vi "check_SQL_statement_type.vi"(7 "SQL_statement_type":T1, 8 "error_in":errorcluster, 11 "SQL_statement_in":string) -> (0 "error_out":errorcluster, 3 "SQL_statement_out":string)   [LabVIEW 2020]
uses:
  SQL_statement_type.ctl
  AULocalize/SubVIs/Get Localized Phrase Compact Interface 0D.vi
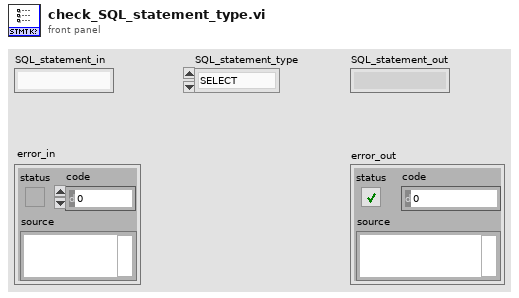
[diagram p1: front panel]
types:
  T1 = typedef "SQL_statement_type.ctl" = enum16{"SELECT", "INSERT", "UPDATE", "DELETE"}
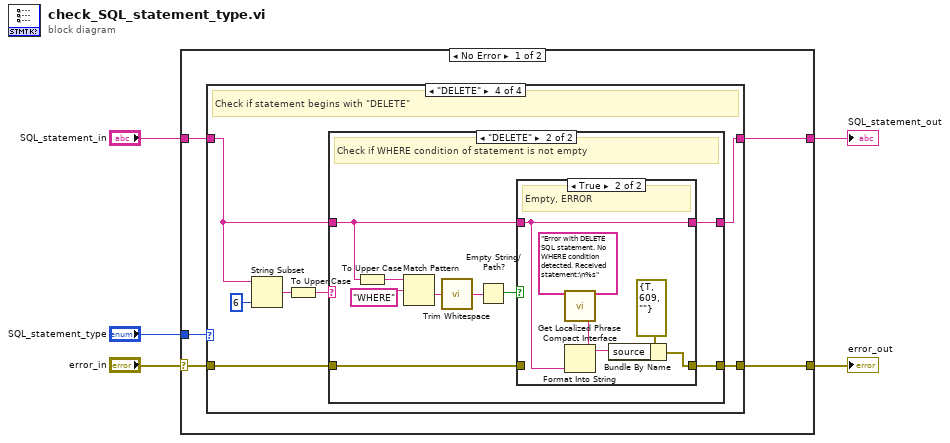
[diagram p0: block diagram]
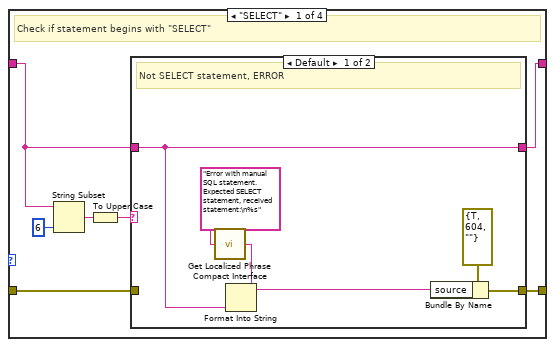
[diagram p2: hidden frame]
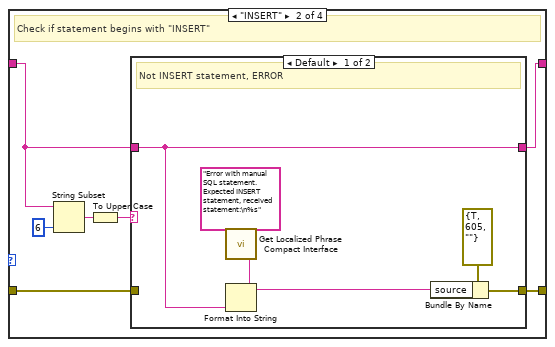
[diagram p4: hidden frame]
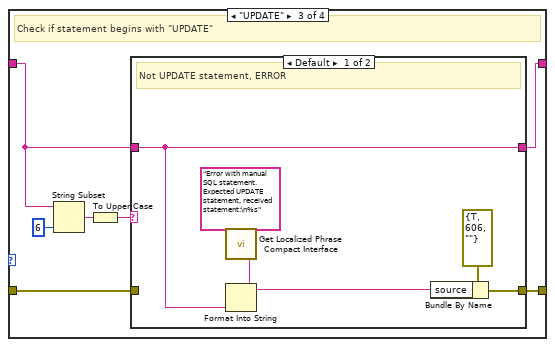
[diagram p6: hidden frame]
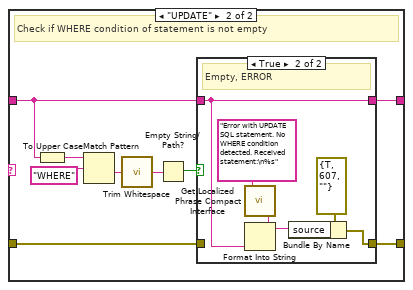
[diagram p7: hidden frame]
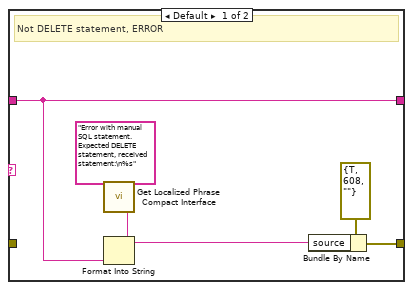
[diagram p9: hidden frame]
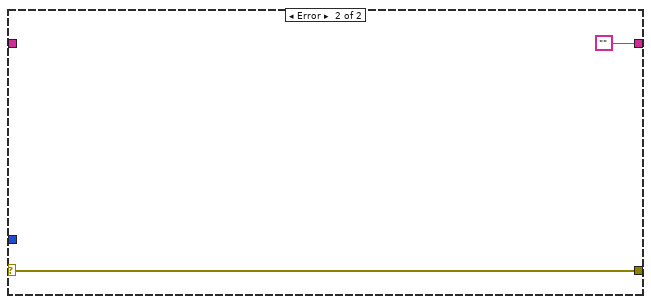
[diagram p11: hidden frame]
diagram:
  n1 = case shown="No Error" "error_in" {
    selector: "error_in" -> [w9 w102]
    tunnel: "SQL_statement_in" -> [w7 _]
    tunnel: [w8 w102] -> w3
    tunnel: "SQL_statement_type" -> [w10 _]
    tunnel: [w6 ""] -> w1
    frame No Error {
      n2 = case shown="\"DELETE\"" w10 {
        tunnel: w7 -> [w14 w29 w44 w74]
        tunnel: w9 -> [w15 w30 w45 w75]
        tunnel: [w16 w31 w46 w76] -> w8
        tunnel: [w11 w26 w41 w71] -> w6
        frame "SELECT" {
          # "Check if statement begins with \"SELECT\""
          n3 = String Subset(string=w14, length (rest)=6 ("length (rest)")) -> (substring=w13:string)  [unwired: 1 in]
          n4 = To Upper Case(1:w13) -> (0:w12:string)
          n5 = case shown="Default" w12 {
            tunnel: [w23 w24] -> w16
            tunnel: w15 -> [_ w24]
            tunnel: w14 -> [w19 w25]
            tunnel: [w19 w25] -> w11
            frame Default {
              # "Not SELECT statement, ERROR"
              n6 = call-poly "Get Localized Phrase Compact Interface.vi"("Key"="Error with manual SQL statement. Expected SELECT statement, received statement:\n%s" ("source")) -> ("Translated Phrase"=w18:string)
              n7 = Format Into String(format string=w18, w19) -> (resulting string=w21:string)  [unwired: 2 in, 1 out]
              n8 = Bundle By Name(cluster=errorcluster {"status"=TRUE, "code"=604, "source"=""} ("error_in"), "source"=w21) -> (w23:errorcluster)
            }
            frame "SELECT" {
              # "SELECT statement, OK"
            }
          }
        }
        frame "INSERT" {
          # "Check if statement begins with \"INSERT\""
          n9 = String Subset(string=w29, length (rest)=6 ("length (rest)")) -> (substring=w28:string)  [unwired: 1 in]
          n10 = To Upper Case(1:w28) -> (0:w27:string)
          n11 = case shown="Default" w27 {
            tunnel: [w38 w39] -> w31
            tunnel: w30 -> [_ w39]
            tunnel: w29 -> [w34 w40]
            tunnel: [w34 w40] -> w26
            frame Default {
              # "Not INSERT statement, ERROR"
              n12 = call-poly "Get Localized Phrase Compact Interface.vi"("Key"="Error with manual SQL statement. Expected INSERT statement, received statement:\n%s" ("source")) -> ("Translated Phrase"=w33:string)
              n13 = Format Into String(format string=w33, w34) -> (resulting string=w36:string)  [unwired: 2 in, 1 out]
              n14 = Bundle By Name(cluster=errorcluster {"status"=TRUE, "code"=605, "source"=""} ("error_in"), "source"=w36) -> (w38:errorcluster)
            }
            frame "INSERT" {
              # "INSERT statement, OK"
            }
          }
        }
        frame "UPDATE" {
          # "Check if statement begins with \"UPDATE\""
          n15 = String Subset(string=w44, length (rest)=6 ("length (rest)")) -> (substring=w43:string)  [unwired: 1 in]
          n16 = To Upper Case(1:w43) -> (0:w42:string)
          n17 = case shown="Default" w42 {
            tunnel: [w53 w56] -> w46
            tunnel: w45 -> [_ w55]
            tunnel: w44 -> [w49 w57]
            tunnel: [w49 w54] -> w41
            frame Default {
              # "Not UPDATE statement, ERROR"
              n18 = call-poly "Get Localized Phrase Compact Interface.vi"("Key"="Error with manual SQL statement. Expected UPDATE statement, received statement:\n%s" ("source")) -> ("Translated Phrase"=w48:string)
              n19 = Format Into String(format string=w48, w49) -> (resulting string=w51:string)  [unwired: 2 in, 1 out]
              n20 = Bundle By Name(cluster=errorcluster {"status"=TRUE, "code"=606, "source"=""} ("error_in"), "source"=w51) -> (w53:errorcluster)
            }
            frame "UPDATE" {
              # "Check if WHERE condition of statement is not empty"
              n21 = To Upper Case(1:w57) -> (0:w60:string)
              n22 = Match Pattern(string=w60, regular expression="WHERE") -> (after substring=w61:string)  [unwired: 1 in, 3 out]
              n23 = call <vilib>:"Trim Whitespace.vi"("string"=w61) -> ("trimmed string"=w59:string)  [unwired: 1 in]
              n24 = Empty String/Path?(string/path=w59) -> (empty?=w58:bool)
              n25 = case shown="True" w58 {
                tunnel: w57 -> [w64 w67]
                tunnel: [w63 w66] -> w56
                tunnel: w55 -> [w63 _]
                tunnel: [w64 w67] -> w54
                frame False {
                  # "Not empty, OK"
                }
                frame True {
                  # "Empty, ERROR"
                  n26 = call-poly "Get Localized Phrase Compact Interface.vi"("Key"="Error with UPDATE SQL statement. No WHERE condition detected. Received statement:\n%s" ("source")) -> ("Translated Phrase"=w65:string)
                  n27 = Format Into String(format string=w65, w67) -> (resulting string=w70:string)  [unwired: 2 in, 1 out]
                  n28 = Bundle By Name(cluster=errorcluster {"status"=TRUE, "code"=607, "source"=""} ("error_in"), "source"=w70) -> (w66:errorcluster)
                }
              }
            }
          }
        }
        frame "DELETE" {
          # "Check if statement begins with \"DELETE\""
          n29 = String Subset(string=w74, length (rest)=6 ("length (rest)")) -> (substring=w73:string)  [unwired: 1 in]
          n30 = To Upper Case(1:w73) -> (0:w72:string)
          n31 = case shown="\"DELETE\"" w72 {
            tunnel: [w83 w86] -> w76
            tunnel: w75 -> [_ w85]
            tunnel: w74 -> [w80 w87]
            tunnel: [w80 w84] -> w71
            frame Default {
              # "Not DELETE statement, ERROR"
              n32 = call-poly "Get Localized Phrase Compact Interface.vi"("Key"="Error with manual SQL statement. Expected DELETE statement, received statement:\n%s" ("source")) -> ("Translated Phrase"=w78:string)
              n33 = Format Into String(format string=w78, w80) -> (resulting string=w81:string)  [unwired: 2 in, 1 out]
              n34 = Bundle By Name(cluster=errorcluster {"status"=TRUE, "code"=608, "source"=""} ("error_in"), "source"=w81) -> (w83:errorcluster)
            }
            frame "DELETE" {
              # "Check if WHERE condition of statement is not empty"
              n35 = To Upper Case(1:w87) -> (0:w90:string)
              n36 = Match Pattern(string=w90, regular expression="WHERE") -> (after substring=w91:string)  [unwired: 1 in, 3 out]
              n37 = call <vilib>:"Trim Whitespace.vi"("string"=w91) -> ("trimmed string"=w89:string)  [unwired: 1 in]
              n38 = Empty String/Path?(string/path=w89) -> (empty?=w88:bool)
              n39 = case shown="True" w88 {
                tunnel: w87 -> [w94 w97]
                tunnel: [w93 w96] -> w86
                tunnel: w85 -> [w93 _]
                tunnel: [w94 w97] -> w84
                frame False {
                  # "Not empty, OK"
                }
                frame True {
                  # "Empty, ERROR"
                  n40 = call-poly "Get Localized Phrase Compact Interface.vi"("Key"="Error with DELETE SQL statement. No WHERE condition detected. Received statement:\n%s" ("source")) -> ("Translated Phrase"=w95:string)
                  n41 = Format Into String(format string=w95, w97) -> (resulting string=w100:string)  [unwired: 2 in, 1 out]
                  n42 = Bundle By Name(cluster=errorcluster {"status"=TRUE, "code"=609, "source"=""} ("error_in"), "source"=w100) -> (w96:errorcluster)
                }
              }
            }
          }
        }
      }
    }
    frame Error {
    }
  }
  "error_out" <- w3
  "SQL_statement_out" <- w1
